vi "test.vi"() -> ()   [LabVIEW 2019]
panel:
  in  "IR sensor":bool
  out "s? t:f":dbl
  in  "Motion sequence or predefined?":bool
  in  "Botton":bool
  in  "Switch mode":bool
  in  "Motion sequence":T1
  out "transposed array":dbl[][](array[numeric])
  out "start position":i32[](array[numeric])
  out "end position":i32[](array[numeric])
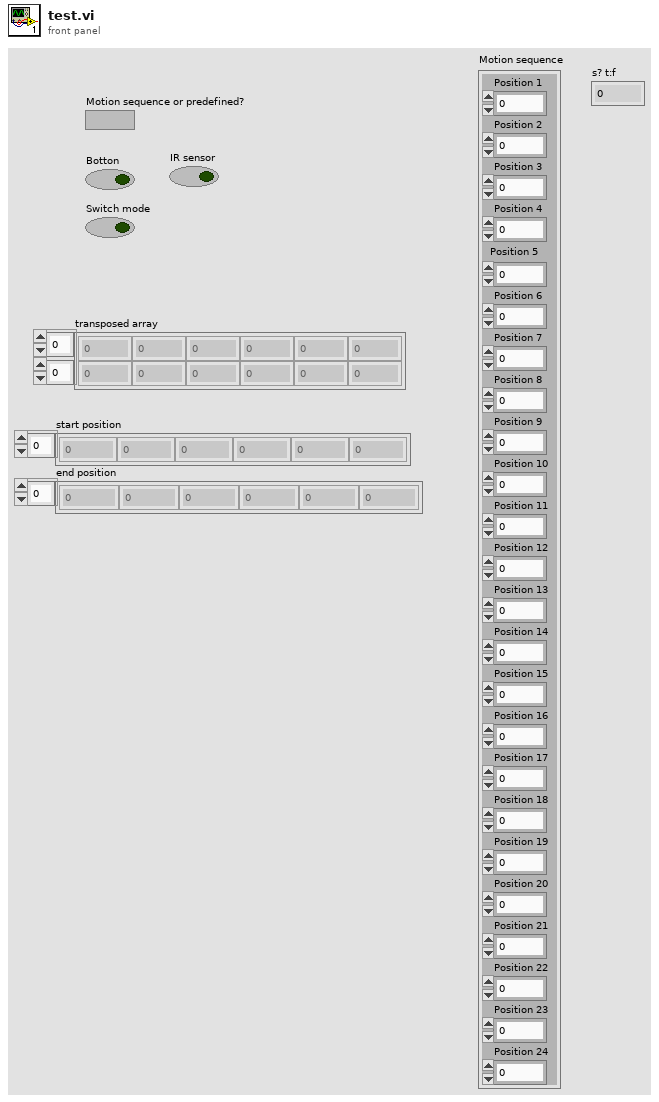
[diagram p1: front panel]
types:
  T1 = cluster{"Position 1":dbl, "Position 2":dbl, "Position 3":dbl, "Position 4":dbl, "Position 5":dbl, "Position 6":dbl, "Position 7":dbl, "Position 8":dbl, "Position 9":dbl, "Position 10":dbl, "Position 11":dbl, "Position 12":dbl, "Position 13":dbl, "Position 14":dbl, "Position 15":dbl, "Position 16":dbl, "Position 17":dbl, "Position 18":dbl, "Position 19":dbl, "Position 20":dbl, "Position 21":dbl, "Position 22":dbl, "Position 23":dbl, "Position 24":dbl}
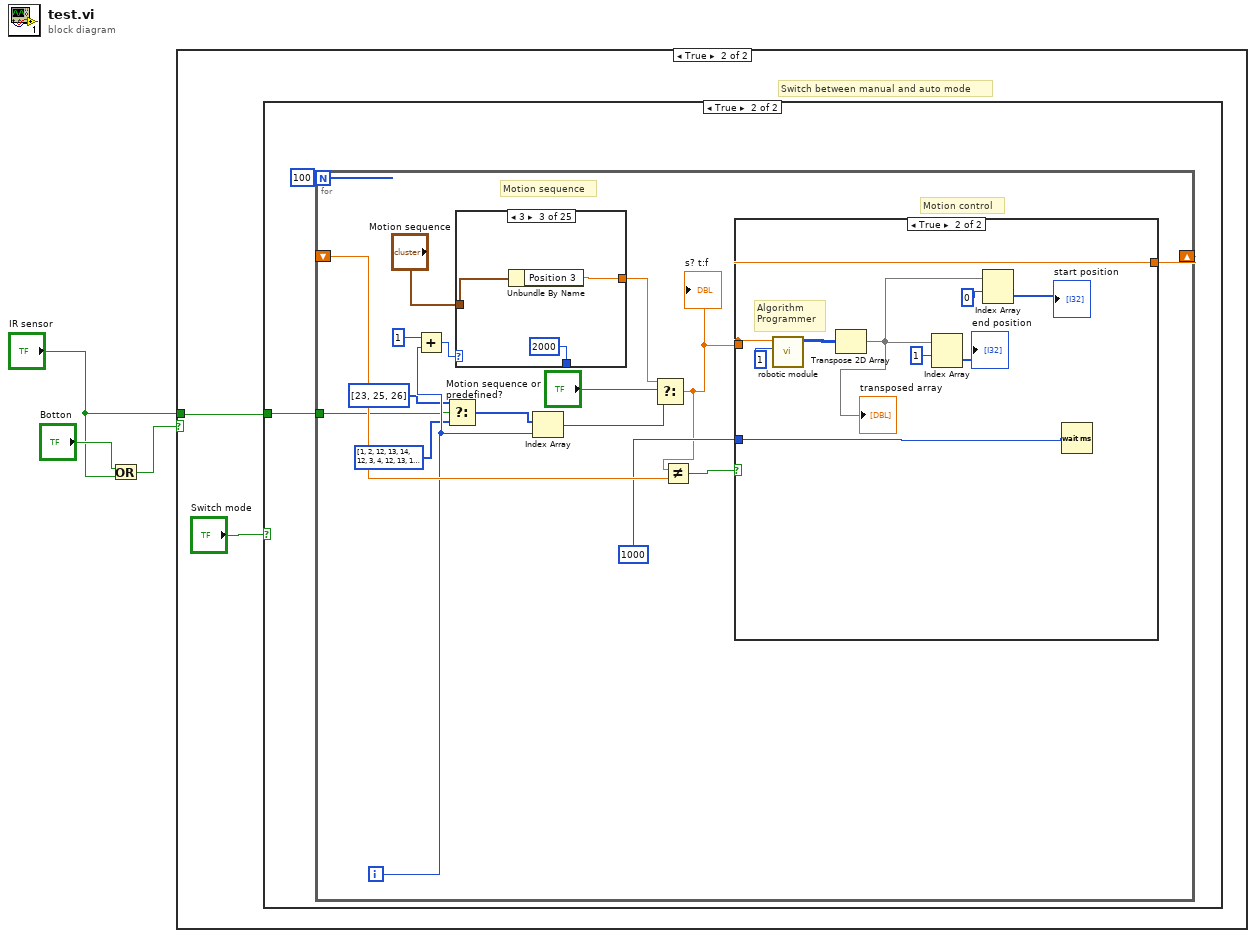
[diagram p0: block diagram]
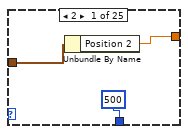
[diagram p4: hidden frame]
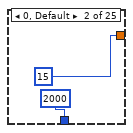
[diagram p5: hidden frame]
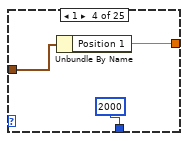
[diagram p6: hidden frame]
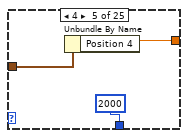
[diagram p7: hidden frame]
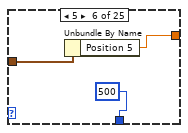
[diagram p8: hidden frame]
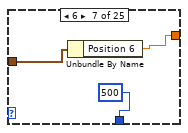
[diagram p9: hidden frame]
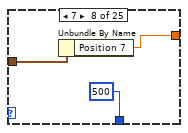
[diagram p10: hidden frame]
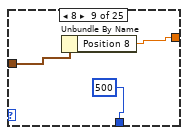
[diagram p11: hidden frame]
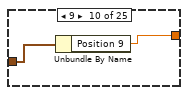
[diagram p12: hidden frame]
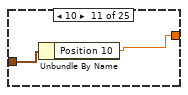
[diagram p13: hidden frame]
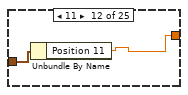
[diagram p14: hidden frame]
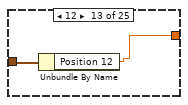
[diagram p15: hidden frame]
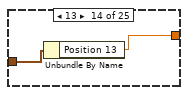
[diagram p16: hidden frame]
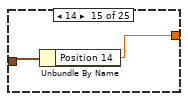
[diagram p17: hidden frame]
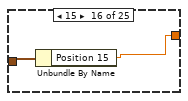
[diagram p18: hidden frame]
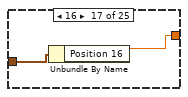
[diagram p19: hidden frame]
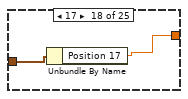
[diagram p20: hidden frame]
diagram:
  n1 = Or(x="Botton", y="IR sensor") -> (x .or. y?=w3:bool)
  n2 = case shown="True" w3 {
    tunnel: "IR sensor" -> [_ w4]
    frame False {
    }
    frame True {
      # "Switch between manual and auto mode"
      n3 = case shown="True" "Switch mode" {
        tunnel: w4 -> [_ w6]
        frame False {
        }
        frame True {
          n4 = for {
            N: 100 -> [_]
            shift-right: [w21] -> _
            shift-left: _ -> [w20]
            tunnel: w6 -> [w9]
            i -> [w14]
            # "Motion control"
            # "Motion sequence"
            n5 = Add(x=1, y=w14) -> (x+y=w12:i32)
            n6 = Select(t=i32[] [23, 25, 26] ("array"), s=w9, f=i32[] [1, 2, 12, 13, 14, 12, 3, 4, 12, 13, 14, 12, 5, 6, 12, 13, 14, 12, 7, 8, 9, 10, 11, 15]) -> (s? t:f=w8:i32[])
            n7 = case shown="3" w12 {
              tunnel: "Motion sequence" -> [w26 _ w31 w34 w36 w40 w42 w46 w47 w50 w52 w54 w56 w58 w61 w62 w64 w66 w68 w70 w72 w74 w76 w79 w80]
              tunnel: [w25 15 w30 w33 w37 w39 w43 w45 w48 w51 w53 w55 w57 w59 w60 w63 w65 w67 w69 w71 w73 w75 w77 w78 w81] -> w18
              tunnel: [u32 500 ("millisecond multiple") u32 2000 ("millisecond multiple") u32 2000 ("millisecond multiple") u32 2000 ("millisecond multiple") u32 2000 ("millisecond multiple") u32 500 ("millisecond multiple") u32 500 ("millisecond multiple") u32 500 ("millisecond multiple") u32 500 ("millisecond multiple") _ _ _ _ _ _ _ _ _ _ _ _ _ _ _ _] -> _
              frame 2 {
                n8 = Unbundle By Name(w26) -> ("Position 2"=w25:dbl)
              }
              frame 0, Default {
              }
              frame 3 {
                n9 = Unbundle By Name(w31) -> ("Position 3"=w30:dbl)
              }
              frame 1 {
                n10 = Unbundle By Name(w34) -> ("Position 1"=w33:dbl)
              }
              frame 4 {
                n11 = Unbundle By Name(w36) -> ("Position 4"=w37:dbl)
              }
              frame 5 {
                n12 = Unbundle By Name(w40) -> ("Position 5"=w39:dbl)
              }
              frame 6 {
                n13 = Unbundle By Name(w42) -> ("Position 6"=w43:dbl)
              }
              frame 7 {
                n14 = Unbundle By Name(w46) -> ("Position 7"=w45:dbl)
              }
              frame 8 {
                n15 = Unbundle By Name(w47) -> ("Position 8"=w48:dbl)
              }
              frame 9 {
                n16 = Unbundle By Name(w50) -> ("Position 9"=w51:dbl)
              }
              frame 10 {
                n17 = Unbundle By Name(w52) -> ("Position 10"=w53:dbl)
              }
              frame 11 {
                n18 = Unbundle By Name(w54) -> ("Position 11"=w55:dbl)
              }
              frame 12 {
                n19 = Unbundle By Name(w56) -> ("Position 12"=w57:dbl)
              }
              frame 13 {
                n20 = Unbundle By Name(w58) -> ("Position 13"=w59:dbl)
              }
              frame 14 {
                n21 = Unbundle By Name(w61) -> ("Position 14"=w60:dbl)
              }
              frame 15 {
                n22 = Unbundle By Name(w62) -> ("Position 15"=w63:dbl)
              }
              frame 16 {
                n23 = Unbundle By Name(w64) -> ("Position 16"=w65:dbl)
              }
              frame 17 {
                n24 = Unbundle By Name(w66) -> ("Position 17"=w67:dbl)
              }
              frame 18 {
                n25 = Unbundle By Name(w68) -> ("Position 18"=w69:dbl)
              }
              frame 19 {
                n26 = Unbundle By Name(w70) -> ("Position 19"=w71:dbl)
              }
              frame 20 {
                n27 = Unbundle By Name(w72) -> ("Position 20"=w73:dbl)
              }
              frame 21 {
                n28 = Unbundle By Name(w74) -> ("Position 21"=w75:dbl)
              }
              frame 22 {
                n29 = Unbundle By Name(w76) -> ("Position 22"=w77:dbl)
              }
              frame 23 {
                n30 = Unbundle By Name(w79) -> ("Position 23"=w78:dbl)
              }
              frame 24 {
                n31 = Unbundle By Name(w80) -> ("Position 24"=w81:dbl)
              }
            }
            n32 = Index Array(array=w8, index=w14) -> (element=w17:i32)
            n33 = Select(t=w18, s="Motion sequence or predefined?", f=w17) -> (s? t:f=w15:dbl)
            "s? t:f" <- w15
            n34 = Not Equal?(x=w15, y=w20) -> (x != y?=w23:bool)
            n35 = case shown="True" w23 {
              tunnel: w15 -> [w82 w86]
              tunnel: [w82 w86] -> w21
              tunnel: u32 1000 ("millisecond multiple") -> [_ w83]
              frame False {
              }
              frame True {
                # "Algorithm\nProgrammer"
                n36 = call "robotic module.vi"("Repeat (MUST BE 1)"=1, "motion type"=w86) -> ("array"=w90:i32[][])  [unwired: 9 in]
                n37 = Transpose 2D Array(2D array=w90) -> (transposed array=w88:i32[][])
                "transposed array" <- w88
                n38 = Index Array(array=w88, index (row)=1) -> (element=→"end position":i32[])  [unwired: 1 in]
                n39 = Index Array(array=w88, index (row)=0) -> (element=→"start position":i32[])  [unwired: 1 in]
                n40 = Wait (ms)(milliseconds to wait=w83) -> ()  [unwired: 1 out]
              }
            }
          }
        }
      }
    }
  }
